vi "Offset Two Points Rectangle.vi"() -> ()   [LabVIEW 2012]
uses:
  demo dll.dll
panel:
  out "OffsetRect":T1
  in  "Point":cluster{"x":i32, "y":i32}
  in  "Rect":T2
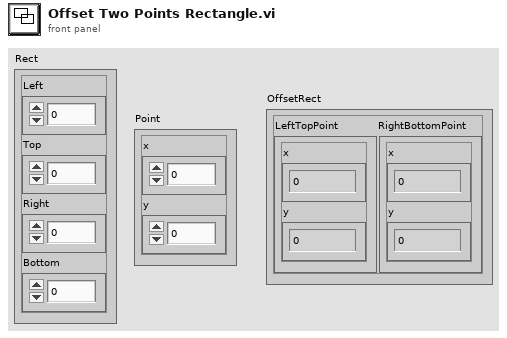
[diagram p1: front panel]
types:
  T1 = cluster{"LeftTopPoint":cluster{"x":i32, "y":i32}, "RightBottomPoint":cluster{"x":i32, "y":i32}}
  T2 = cluster{"Left":i32, "Top":i32, "Right":i32, "Bottom":i32}
  T3 = cluster{"Point":cluster{"x":i32, "y":i32}, "Point":cluster{"x":i32, "y":i32}}
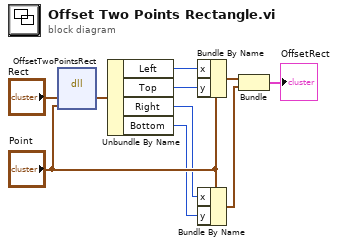
[diagram p0: block diagram]
diagram:
  n1 = dll-call lib="PTH1+abs EBOOK\t功能块DLLdemo dll.dll" fn="OffsetTwoPointsRect"("Rect"="Rect", "OffPoint"="Point") -> ("Rect"=w9:T2)  [unwired: 5 in, 2 out]
  n2 = Unbundle By Name(w9) -> ("Left"=w8:i32, "Top"=w6:i32, "Right"=w5:i32, "Bottom"=w4:i32)
  n3 = Bundle By Name(cluster="Point", "x"=w8, "y"=w6) -> (w3:cluster{"x":i32, "y":i32})
  n4 = Bundle By Name(cluster="Point", "x"=w5, "y"=w4) -> (w2:cluster{"x":i32, "y":i32})
  n5 = Bundle("Point"=w3, "Point"=w2) -> (→"OffsetRect":T3)  [unwired: 1 in]
